vi "RSZVB Auto Length.vi"(8 "error in (no error)":errorcluster {"code" format="%.0x"}, 9 "Port (1)":i32=1, 10 "Channel (1)":i32=1, 11 "VISA session":refnum<visa-resource-name>) -> (0 "error out":errorcluster {"code" format="%.0x"}, 3 "dup VISA session":refnum<visa-resource-name>)   [LabVIEW 2011]
doc: "This VI defines the offset parameter for the active test port such that the residual delay of the active trace is minimized across the entire sweep range.\n\nNote(s):\n\nRemote-control command(s):\n[SENSe<Ch>:]CORRection:EDELay<port_no>:AUTO ONCE"
uses:
  _utility/RSZVB Global Data.vi
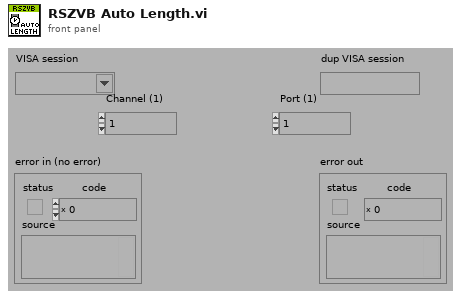
[diagram p1: front panel]
types:
  T1 = cluster{"Error Checking (T: On)":bool, "Installed Options":string[], "Data Valid?":bool, "Ports":i32, "Model":string[], "Option Checking (T: On)":bool}[]
  T2 = cluster{"Error Checking (T: On)":bool, "Installed Options":string[], "Data Valid?":bool, "Ports":i32, "Model":string[], "Option Checking (T: On)":bool}
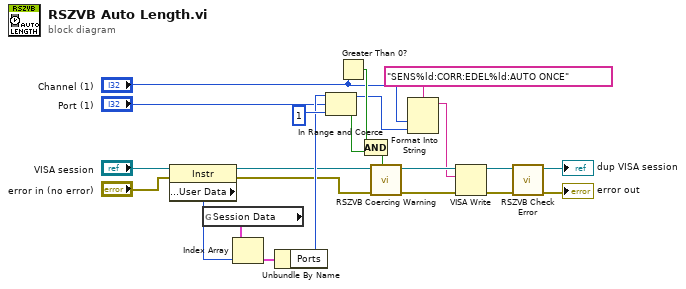
[diagram p0: block diagram]
diagram:
  n1 = property class="Instr"(reference="VISA session", error in="error in (no error)") -> (reference out=w9:refnum<visa-resource-name>, error out=w10:errorcluster, "General Settings:User Data"=w13:u32)
  n2 = global read "RSZVB Global Data.vi" "Session Data"() -> (w14:T1)
  n3 = Index Array(array=w14, index=w13) -> (element=w15:T2)
  n4 = Unbundle By Name(w15) -> ("Ports"=w11:i32)
  n5 = In Range and Coerce(upper limit=w11, x="Port (1)", lower limit=1) -> (coerced(x)=w8:i32, In Range?=w7:bool)
  n6 = Greater Than 0?(x="Channel (1)") -> (x > 0?=w16:bool)
  n7 = Compound Arithmetic op=AND(w16, w7) -> (w18:bool)
  n8 = call "RSZVB Coercing Warning.vi"("In Range?"=w18, "error in (no error)"=w10, "VISA session"=w9) -> ("error out"=w21:errorcluster, "dup VISA session"=w22:refnum<visa-resource-name>)  [unwired: 7 in]
  n9 = Format Into String(format string="SENS%ld:CORR:EDEL%ld:AUTO ONCE", "Channel (1)", w8) -> (resulting string=w17:string)  [unwired: 2 in, 1 out]
  n10 = VISA Write(VISA resource name=w22, write buffer=w17, error in (no error)=w21) -> (VISA resource name out=w19:refnum<visa-resource-name>, error out=w20:errorcluster)  [unwired: 1 out]
  n11 = call "RSZVB Check Error.vi"("error in (no error)"=w20, "VISA session"=w19) -> ("error out"=→"error out":errorcluster, "dup VISA session"=→"dup VISA session":refnum<visa-resource-name>)  [unwired: 8 in]
